vi "Add Resource (IQ Data Trigger).vi"(0 "instance":u8, 1 "trigger type":T1, 2 "acq in":refnum<class "niUSRP DSP v2 FPGA.lvclass">=refnum, 3 "collection builder in":refnum<class "Collection Builder.lvclass">=refnum, 5 "IP enabled":bool) -> (13 "acq out":refnum<class "niUSRP DSP v2 FPGA.lvclass">, 14 "collection builder out":refnum<class "Collection Builder.lvclass">)   [LabVIEW 2023]
uses:
  <instrlib>/_niInstr/DSP Control/Interface/v1/FPGA/IQ Data Trigger/IQ 18-bit/IQ Data Trigger Interface (18-bit).lvclass
  <instrlib>/_niInstr/DSP Control/Common/v2/FPGA/IQ Data Trigger/Registers (IQ 18-bit)/IQ Data Trigger Type.ctl
  <instrlib>/niVST/Reference FPGA/FPGA/ACQ DSP/niUSRP DSP v2 FPGA.lvclass
  <instrlib>/_niInstr/Instruction Framework/v1/FPGA/Collection Builder/Collection Builder.lvclass
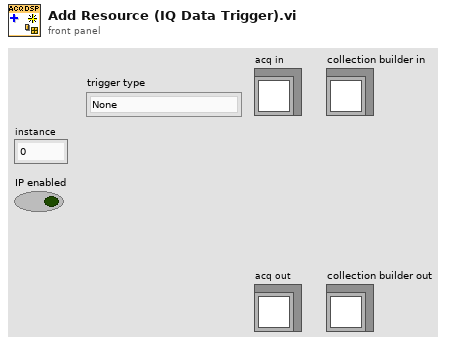
[diagram p1: front panel]
types:
  T1 = typedef "niInstr DSP Control Common v2 FPGA.lvlib/IQ Data Trigger Registers (IQ 18-bit).lvclass/IQ Data Trigger Type.ctl" = enum8{"None", "Power Edge", "Analog Edge", "Analog and Power Edge"}
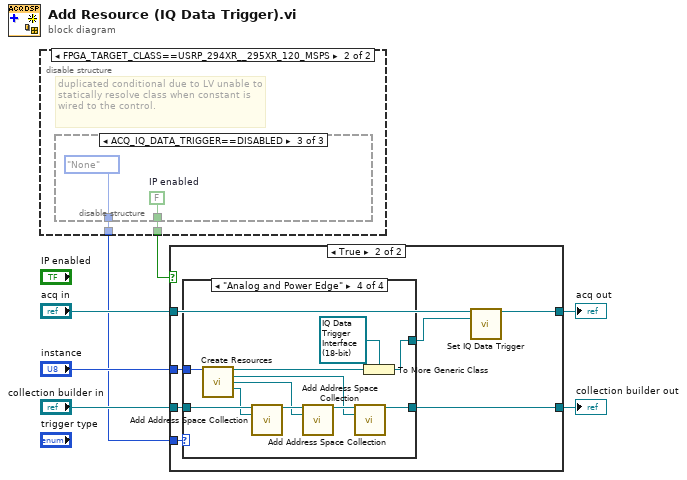
[diagram p0: block diagram]
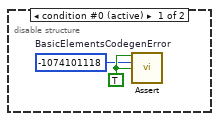
[diagram p2: hidden frame]
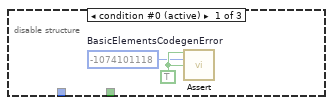
[diagram p3: hidden frame]
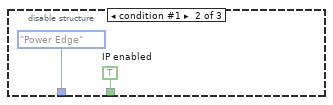
[diagram p4: hidden frame]
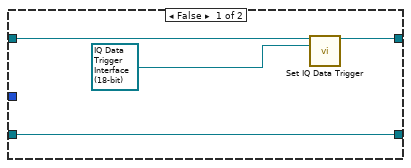
[diagram p5: hidden frame]
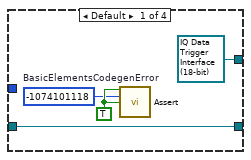
[diagram p6: hidden frame]
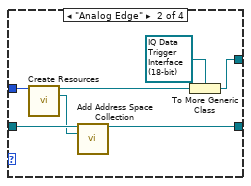
[diagram p7: hidden frame]
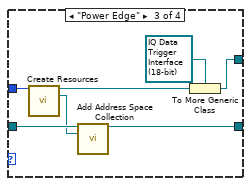
[diagram p8: hidden frame]
diagram:
  n1 = disable-structure shown="FPGA_TARGET_CLASS==USRP_294XR__295XR_120_MSPS" {
    disable-tunnel: [_ w11] -> w2
    disable-tunnel: [_ w10] -> w1
    frame condition #0 (active) {
      w9 = TRUE ("assert")
      w8 = -1074101118  # BasicElementsCodegenError
      n2 = call <instrlib>:"Assert.vi"("assert"=w9, "error code"=w8, "enable show error"=w9) -> ()  [unwired: 13 in]
    }
    frame condition #1 {
      # "duplicated conditional due to LV unable to statically resolve class when constant is wired to the control."
      n3 = disable-structure shown="ACQ_IQ_DATA_TRIGGER==DISABLED" {
        disable-tunnel: [_ w15 w16] -> w11
        disable-tunnel: [_ IQ_Data_Trigger_Type."Power Edge" ("trigger type") IQ_Data_Trigger_Type."None" ("trigger type")] -> w10
        frame condition #0 (active) {
          w13 = TRUE ("assert")
          w12 = -1074101118  # BasicElementsCodegenError
          n4 = call <instrlib>:"Assert.vi"("assert"=w13, "error code"=w12, "enable show error"=w13) -> ()  [unwired: 13 in]
        }
        frame condition #1 {
          w15 = TRUE  # IP enabled
        }
        frame condition #2 {
          w16 = FALSE  # IP enabled
        }
      }
    }
  }
  n5 = case shown="True" w2 {
    tunnel: "collection builder in" -> [w21 w28]
    tunnel: [w21 w27] -> w6
    tunnel: "instance" -> [_ w26]
    tunnel: "acq in" -> [w19 w24]
    tunnel: [w18 w23] -> w3
    tunnel: w1 -> [_ w25]
    frame False {
      n6 = call-dynamic "Set IQ Data Trigger.vi"("acq in"=w19, "iq data trigger"=refnum<class "IQ Data Trigger Interface (18-bit).lvclass"> refnum ("iq impairments")) -> ("acq out"=w18:refnum<class "niUSRP DSP v2 FPGA.lvclass">)  [unwired: 13 in]
    }
    frame True {
      n7 = case shown="\"Analog and Power Edge\"" w25 {
        tunnel: w28 -> [w31 w39 w46 w57]
        tunnel: [w31 w38 w45 w50] -> w27
        tunnel: w26 -> [_ w37 w44 w56]
        tunnel: [refnum<class "IQ Data Trigger Interface (18-bit).lvclass"> refnum ("iq data trigger") w33 w40 w53] -> w22
        frame Default {
          w30 = TRUE ("assert")
          w29 = -1074101118  # BasicElementsCodegenError
          n8 = call <instrlib>:"Assert.vi"("assert"=w30, "error code"=w29, "enable show error"=w30) -> ()  [unwired: 13 in]
        }
        frame "Analog Edge" {
          n9 = call <instrlib>:"Create Resources.vi"("instance"=w37) -> ("iq analog edge"=w34:refnum<class "IQ Analog Edge Trigger (IQ 18-bit).lvclass">, "iq analog edge registers"=w36:refnum<class "Single Address Space Collection.lvclass">)  [unwired: 13 in]
          n10 = call <instrlib>:"Add Address Space Collection.vi"("collection builder in"=w39, "address space collection"=w36) -> ("collection builder out"=w38:refnum<class "Collection Builder.lvclass">)  [unwired: 13 in]
          n11 = To More Generic Class(target class=refnum<class "IQ Data Trigger Interface (18-bit).lvclass"> refnum ("iq data trigger"), reference=w34) -> (generic class reference=w33:refnum<class "IQ Data Trigger Interface (18-bit).lvclass">)
        }
        frame "Power Edge" {
          n12 = call <instrlib>:"Create Resources.vi"("instance"=w44) -> ("iq power edge"=w41:refnum<class "IQ Power Edge Trigger (IQ 18-bit).lvclass">, "iq power edge registers"=w43:refnum<class "Single Address Space Collection.lvclass">)  [unwired: 13 in]
          n13 = call <instrlib>:"Add Address Space Collection.vi"("collection builder in"=w46, "address space collection"=w43) -> ("collection builder out"=w45:refnum<class "Collection Builder.lvclass">)  [unwired: 13 in]
          n14 = To More Generic Class(target class=refnum<class "IQ Data Trigger Interface (18-bit).lvclass"> refnum ("iq data trigger"), reference=w41) -> (generic class reference=w40:refnum<class "IQ Data Trigger Interface (18-bit).lvclass">)
        }
        frame "Analog and Power Edge" {
          n15 = call <instrlib>:"Create Resources.vi"("instance"=w56) -> ("iq anlg and pow"=w54:refnum<class "IQ Analog and Power Edge Trigger (IQ 18-bit).lvclass">, "iq anlg and pow registers"=w47:refnum<class "Single Address Space Collection.lvclass">, "iq analog edge registers"=w48:refnum<class "Single Address Space Collection.lvclass">, "iq power edge registers"=w49:refnum<class "Single Address Space Collection.lvclass">)  [unwired: 11 in]
          n16 = call <instrlib>:"Add Address Space Collection.vi"("collection builder in"=w57, "address space collection"=w49) -> ("collection builder out"=w52:refnum<class "Collection Builder.lvclass">)  [unwired: 13 in]
          n17 = call <instrlib>:"Add Address Space Collection.vi"("collection builder in"=w52, "address space collection"=w48) -> ("collection builder out"=w51:refnum<class "Collection Builder.lvclass">)  [unwired: 13 in]
          n18 = call <instrlib>:"Add Address Space Collection.vi"("collection builder in"=w51, "address space collection"=w47) -> ("collection builder out"=w50:refnum<class "Collection Builder.lvclass">)  [unwired: 13 in]
          n19 = To More Generic Class(target class=refnum<class "IQ Data Trigger Interface (18-bit).lvclass"> refnum ("iq data trigger"), reference=w54) -> (generic class reference=w53:refnum<class "IQ Data Trigger Interface (18-bit).lvclass">)
        }
      }
      n20 = call-dynamic "Set IQ Data Trigger.vi"("acq in"=w24, "iq data trigger"=w22) -> ("acq out"=w23:refnum<class "niUSRP DSP v2 FPGA.lvclass">)  [unwired: 13 in]
    }
  }
  "collection builder out" <- w6
  "acq out" <- w3
